vi "writeToXML.vi"(8 "error in (no error)":errorcluster, 10 "classLabel":string, 11 "GuideAutoclearState in":refnum<class "GuideAutoclearState.lvclass">) -> (0 "error out":errorcluster, 2 "XML out":string, 3 "GuideAutoclearState out":refnum<class "GuideAutoclearState.lvclass">)   [LabVIEW 2022 SP3, in "TCSDataDefinitions.lvlib" / "TCSCommand.lvlib" / "GuiderCommands.lvlib" / "GuideAutoclearState.lvclass"]
uses:
  GuideAutoclearState.lvclass
  GuideAutoclearState.lvclass/GuideAutoclearState.ctl
  GuiderCommands.lvclass
  <userlib>/Common/XML/XMLGenerator/XMLGenerator.lvclass
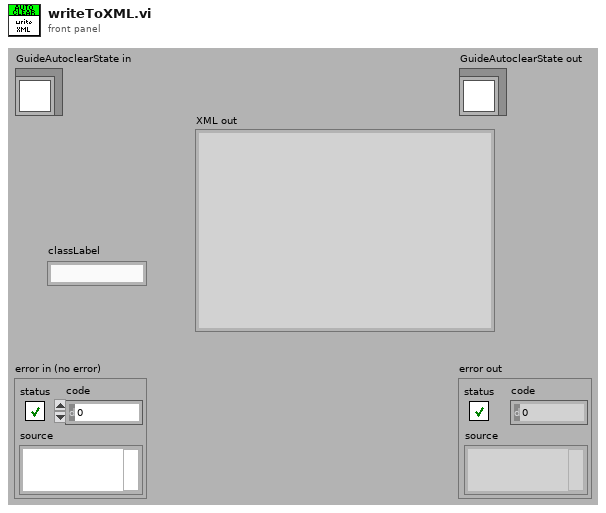
[diagram p1: front panel]
types:
  T1 = typedef "TCSDataDefinitions.lvlib/TCSCommand.lvlib/GuideAutoclearStateTypes.ctl" = enum16{"On", "Off"}
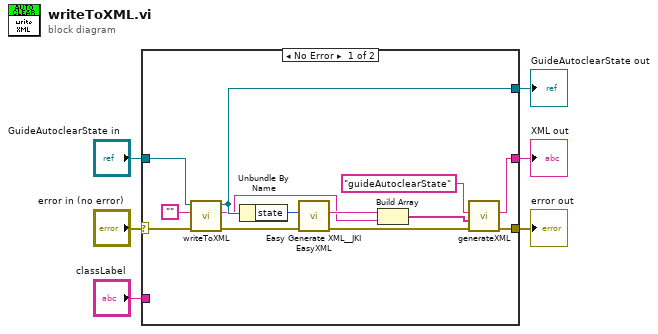
[diagram p0: block diagram]
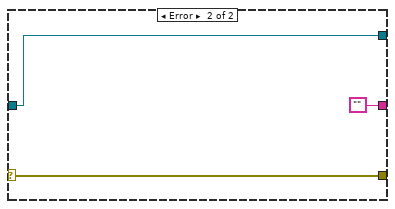
[diagram p2: hidden frame]
diagram:
  n1 = case shown="No Error" "error in (no error)" {
    selector: "error in (no error)" -> [w8 w22]
    tunnel: [w7 w22] -> w5
    tunnel: [w17 w21] -> w3
    tunnel: "GuideAutoclearState in" -> [w19 w21]
    tunnel: [w9 ""] -> w2
    tunnel: "classLabel" -> [_ _]
    frame No Error {
      n2 = call-parent "writeToXML.vi"("error in (no error)"=w8, "ClassLabel"="", "GuiderCommands in"=w19) -> ("error out"=w15:errorcluster, "XML out"=w13:string, "GuiderCommands out"=w17:refnum<class "GuideAutoclearState.lvclass">)  [unwired: 6 in]
      n3 = Unbundle By Name(w17) -> ("state"=w16:T1)
      n4 = call <vilib>:"Easy Generate XML__JKI EasyXML.vi"("error in (no error)"=w15, "LabVIEW Data"=w16) -> ("error out"=w12:errorcluster, "XML String"=w14:string)  [unwired: 8 in]
      n5 = Build Array(w14, w13) -> (w11:string[])
      n6 = call <userlib>:"generateXML.vi"("error in"=w12, "childrenXML"=w11, "elementName"="guideAutoclearState" ("Class Label")) -> ("error out"=w7:errorcluster, "XML out"=w9:string)  [unwired: 6 in, 1 out]
    }
    frame Error {
    }
  }
  "error out" <- w5
  "GuideAutoclearState out" <- w3
  "XML out" <- w2
